vi "Waveform Cluster (2D) to Spreadsheet String.vi"(1 "waveform cluster":cluster{i32, "dx":dbl, "Array":dbl[][]}) -> (0 "spreadsheet string":string)   [LabVIEW 2020]
uses:
  Math VIs/LinSpace (x0-dx-npts).vi
  Array Manipulation VIs/Array-Dimensions (2D).vi
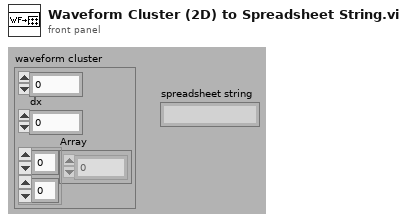
[diagram p1: front panel]
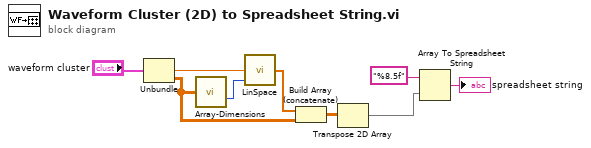
[diagram p0: block diagram]
diagram:
  n1 = Unbundle("waveform cluster") -> ("dx"=w8:dbl, "Array"=w2:dbl[][])  [unwired: 1 out]
  n2 = call-poly "Array-Dimensions.vi"("2D Array"=w2) -> ("# columns"=w1:i32)  [unwired: 13 in, 1 out]
  n3 = call-poly "LinSpace.vi"("npts"=w1, "dx"=w8) -> ("Array"=w6:dbl[])  [unwired: 2 in, 1 out]
  n4 = Build Array (concatenate)(w6, w2) -> (w5:dbl[][])
  n5 = Transpose 2D Array(2D array=w5) -> (transposed array=w4:dbl[][])
  n6 = Array To Spreadsheet String(array=w4, 3:"%8.5f" ("format (%.3f)")) -> (spreadsheet string=→"spreadsheet string":string)  [unwired: 1 in]
